vi "AB_Get_Skip_Icon_Token.vi"(8 "error in (no error)":errorcluster) -> (0 "error out":errorcluster, 3 "skipIconLoad":bool)   [LabVIEW 2020]
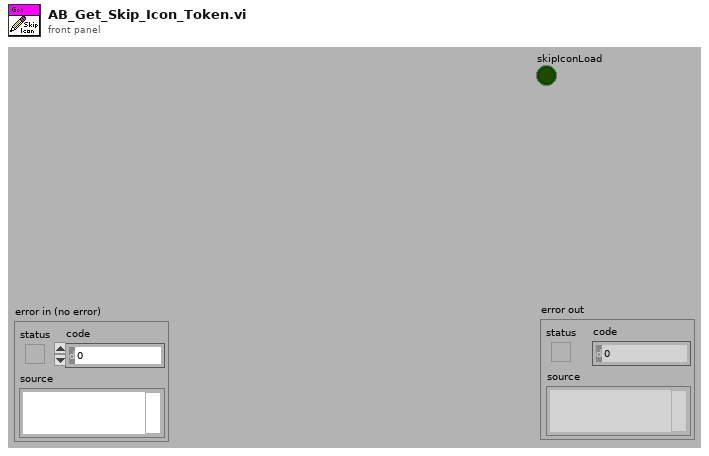
[diagram p1: front panel]
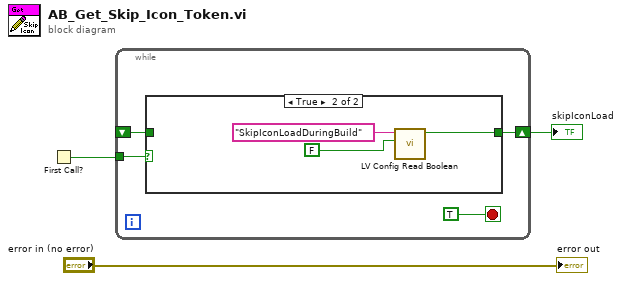
[diagram p0: block diagram]
diagram:
  n1 = First Call?() -> (First Call?: T/F=w1:bool)
  n2 = while {
    shift-right: [w6] -> w2
    shift-left: _ -> [w4]
    tunnel: w1 -> [w5]
    stop <- TRUE stop-if-true
    n3 = case shown="True" w5 {
      tunnel: [w8 w11] -> w6
      tunnel: w4 -> [w8 _]
      frame False {
      }
      frame True {
        n4 = call <resource>:"LV Config Read Boolean.vi"("default value"=FALSE, "key"="SkipIconLoadDuringBuild") -> ("value"=w11:bool)  [unwired: 1 in, 4 out]
      }
    }
  }
  "skipIconLoad" <- w2
  "error out" <- "error in (no error)"
